vi "CRYReport Check.vi"() -> (2 "bResult":bool)   [LabVIEW 2013]
panel:
  in  "TXButtonBar":refnum<k7>(container)
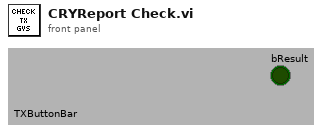
[diagram p1: front panel]
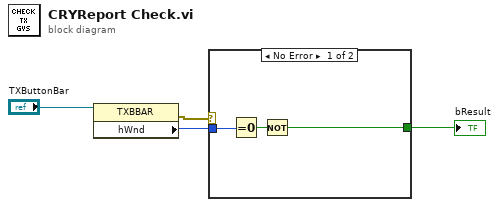
[diagram p0: block diagram]
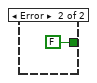
[diagram p2: hidden frame]
diagram:
  n1 = property class="TXBBAR"(reference="TXButtonBar") -> (error out=w2:errorcluster, "hWnd"=w4:i32)  [unwired: 1 in, 1 out]
  n2 = case shown="No Error" w2 {
    tunnel: w4 -> [w7 _]
    tunnel: [w5 FALSE] -> w1
    frame No Error {
      n3 = Equal To 0?(x=w7) -> (x = 0?=w6:bool)
      n4 = Not(x=w6) -> (.not. x?=w5:bool)
    }
    frame Error {
    }
  }
  "bResult" <- w1
